vi "Change Bits (I64).vi"(9 "Values":bool[](array[boolean]), 10 "Bits":u8[](array[numeric]), 11 "Number":i64 format="%.0x") -> (3 "Number Out":i64 format="%.0x")   [LabVIEW 2019, in "Bits.lvlib"]
doc: "Changes the bits in the passed in number to the specified values."
uses:
  Bits.lvlib
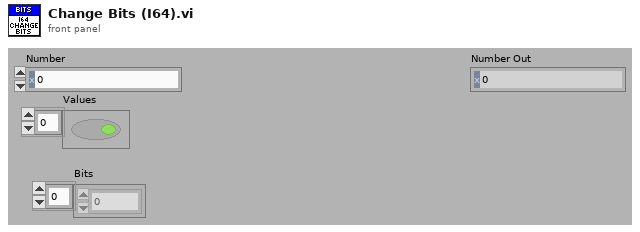
[diagram p1: front panel]
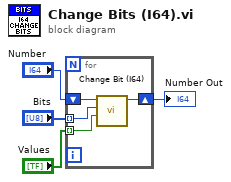
[diagram p0: block diagram]
diagram:
  n1 = for {
    shift-right: [w7] -> w4
    shift-left: "Number" -> [w8]
    tunnel: "Bits" -> [w6] mode=indexing
    tunnel: "Values" -> [w5] mode=indexing
    n2 = call "Change Bit (I64).vi"("Value"=w5, "Bit"=w6, "Number"=w8) -> ("Number Out"=w7:i64)  [unwired: 8 in]
  }
  "Number Out" <- w4
